vi "Get Current Branch Status.vi"(8 "error in (no error)":errorcluster, 11 "abs_Parallel in":refnum<class "bt_Parallel.lvclass">) -> (0 "error out":errorcluster, 2 "Previous Status":T1, 3 "abs_Parallel out":refnum<class "bt_Parallel.lvclass">)   [LabVIEW 2021, in "BT.lvlib" / "bt_Parallel.lvclass"]
uses:
  bt_Parallel.lvclass
  C:/Users/Tim/Documents/GitHub/LV_Behaviour_Tree/Source/Support/Nodes/Composites/abs_Composite/bt_Composite.lvclass
  abs_Node/Status.ctl
  abs_Composite/bt_Composite.lvclass/bt_Composite.ctl
  bt_Parallel.lvclass/bt_Parallel.ctl
  abs_Composite/Properties/Read Index.vi
  abs_Node/bt_Node.lvclass
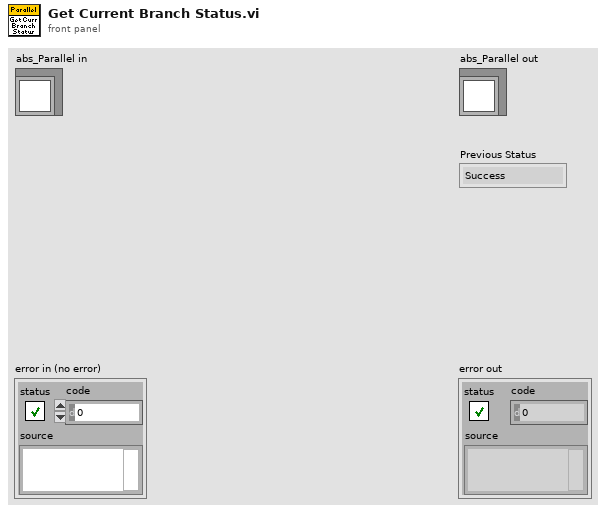
[diagram p1: front panel]
types:
  T1 = typedef "BT.lvlib/bt_Node.lvclass/Status.ctl" = enum16{"Success", "Failure", "Running"}
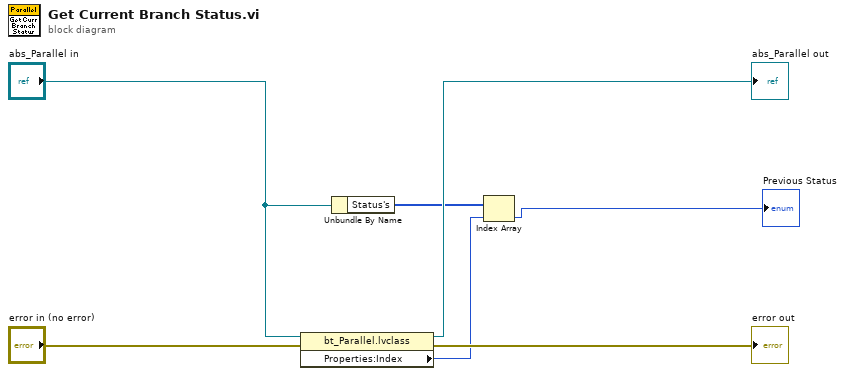
[diagram p0: block diagram]
diagram:
  n1 = property class="bt_Parallel.lvclass"(reference="abs_Parallel in", error in="error in (no error)") -> (reference out=→"abs_Parallel out":refnum<class "bt_Parallel.lvclass">, error out=→"error out":errorcluster, "Properties:Index"=w1:i32)
  n2 = Unbundle By Name("abs_Parallel in") -> ("Status's"=w2:T1[])
  n3 = Index Array(array=w2, index=w1) -> (element=→"Previous Status":T1)
